vi "Configure Maximum File Size.vi"(8 "Error In":errorcluster, 11 "File Size":i32=15728640) -> (0 "Error Out":errorcluster)   [LabVIEW 2017, in "Toolkit.lvlib"]
doc: "Sets the maximum file size for the default log file before initiating a rollover event, where a new log file is created automatically. If the current log file size is greater or equal to this value after writing the previous logging statement, then the file is closed and a new log file is created. The new log file will have a file name using the ISO 8601 timestamp format."
uses:
  Toolkit.lvlib
  Support VIs/File/Action.ctl
  Support VIs/File/File.lvlib
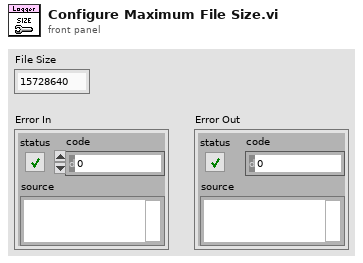
[diagram p1: front panel]
types:
  T1 = typedef "Toolkit.lvlib/File.lvlib/Action.ctl" = enum16{"Initialize", "Set Maximum File Size", "Set Maximum File Count", "Set Root Folder", "Set Enable Calendar Folder Tree", "Set File Extension", "Start", "Write", "Stop", "Shutdown"}
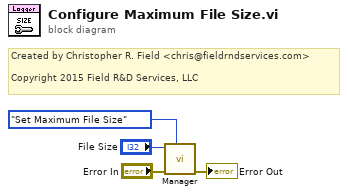
[diagram p0: block diagram]
diagram:
  # "Created by Christopher R. Field <chris@fieldrndservices.com>\n\nCopyright 2015 Field R&D Services, LLC"
  n1 = call "Manager.vi"("Action"=Action."Set Maximum File Size", "Error In"="Error In", "Set Value"="File Size") -> ("Error Out"=→"Error Out":errorcluster)  [unwired: 8 in]
